vi "GetProbePlanCoordinates.vi"(8 "Use index as X coord":bool=TRUE, 9 "Probe Card Channels":i32=1) -> (0 "file path":string, 2 "OK?":bool, 3 "Array":T1(array[cluster]))   [LabVIEW 2018] (continued)
557\tX=44004.84\ty=-3214.74 \nLabel=Strip\t558\tX=44355.35\ty=-3136.62 \nLabel=Strip\t559\tX=44005.91\ty=-3067.71 \nLabel=Strip\t560\tX=44356.40\ty=-2989.46 \nLabel=Strip\t561\tX=44006.94\ty=-2920.67 \nLabel=Strip\t562\tX=44357.40\ty=-2842.30 \nLabel=Strip\t563\tX=44007.92\ty=-2773.62 \nLabel=Strip\t564\tX=44358.36\ty=-2695.14 \nLabel=Strip\t565\tX=44008.85\ty=-2626.58 \nLabel=Strip\t566\tX=44359.26\ty=-2547.98 \nLabel=Strip\t567\tX=44009.72\ty=-2479.54 \nLabel=Strip\t568\tX=44360.11\ty=-2400.81 \nLabel=Strip\t569\tX=44010.55\ty=-2332.49 \nLabel=Strip\t570\tX=44360.90\ty=-2253.65 \nLabel=Strip\t571\tX=44011.33\ty=-2185.45 \nLabel=Strip\t572\tX=44361.65\ty=-2106.48 \nLabel=Strip\t573\tX=44012.05\ty=-2038.40 \nLabel=Strip\t574\tX=44362.35\ty=-1959.31 \nLabel=Strip\t575\tX=44012.73\ty=-1891.35 \nLabel=Strip\t576\tX=44363.00\ty=-1812.14 \nLabel=Strip\t577\tX=44013.35\ty=-1744.30 \nLabel=Strip\t578\tX=44363.60\ty=-1664.97 \nLabel=Strip\t579\tX=44013.93\ty=-1597.25 \nLabel=Strip\t580\tX=44364.14\ty=-1517.80 \nLabel=Strip\t581\tX=44014.45\ty=-1450.20 \nLabel=Strip\t582\tX=44364.64\ty=-1370.62 \nLabel=Strip\t583\tX=44014.92\ty=-1303.14 \nLabel=Strip\t584\tX=44365.08\ty=-1223.45 \nLabel=Strip\t585\tX=44015.34\ty=-1156.09 \nLabel=Strip\t586\tX=44365.48\ty=-1076.27 \nLabel=Strip\t587\tX=44015.72\ty=-1009.03 \nLabel=Strip\t588\tX=44365.82\ty=-929.10 \nLabel=Strip\t589\tX=44016.04\ty=-861.97 \nLabel=Strip\t590\tX=44366.12\ty=-781.92 \nLabel=Strip\t591\tX=44016.31\ty=-714.91 \nLabel=Strip\t592\tX=44366.36\ty=-634.74 \nLabel=Strip\t593\tX=44016.53\ty=-567.86 \nLabel=Strip\t594\tX=44366.55\ty=-487.56 \nLabel=Strip\t595\tX=44016.70\ty=-420.79 \nLabel=Strip\t596\tX=44366.70\ty=-340.38 \nLabel=Strip\t597\tX=44016.82\ty=-273.73 \nLabel=Strip\t598\tX=44366.79\ty=-193.19 \nLabel=Strip\t599\tX=44016.89\ty=-126.67 \nLabel=Strip\t600\tX=44366.83\ty=-46.01 \nLabel=Strip\t601\tX=44016.90\ty=20.39 \nLabel=Strip\t602\tX=44366.82\ty=101.17 \nLabel=Strip\t603\tX=44016.87\ty=167.46 \nLabel=Strip\t604\tX=44366.76\ty=248.36 \nLabel=Strip\t605\tX=44016.79\ty=314.53 \nLabel=Strip\t606\tX=44366.65\ty=395.55 \nLabel=Strip\t607\tX=44016.66\ty=461.59 \nLabel=Strip\t608\tX=44366.49\ty=542.73 \nLabel=Strip\t609\tX=44016.47\ty=608.66 \nLabel=Strip\t610\tX=44366.28\ty=689.92 \nLabel=Strip\t611\tX=44016.24\ty=755.73 \nLabel=Strip\t612\tX=44366.01\ty=837.11 \nLabel=Strip\t613\tX=44015.95\ty=902.80 \nLabel=Strip\t614\tX=44365.70\ty=984.30 \nLabel=Strip\t615\tX=44015.62\ty=1049.87 \nLabel=Strip\t616\tX=44365.34\ty=1131.49 \nLabel=Strip\t617\tX=44015.23\ty=1196.94 \nLabel=Strip\t618\tX=44364.92\ty=1278.69 \nLabel=Strip\t619\tX=44014.80\ty=1344.01 \nLabel=Strip\t620\tX=44364.46\ty=1425.88 \nLabel=Strip\t621\tX=44014.31\ty=1491.09 \nLabel=Strip\t622\tX=44363.94\ty=1573.07 \nLabel=Strip\t623\tX=44013.77\ty=1638.16 \nLabel=Strip\t624\tX=44363.38\ty=1720.27 \nLabel=Strip\t625\tX=44013.18\ty=1785.24 \nLabel=Strip\t626\tX=44362.76\ty=1867.46 \nLabel=Strip\t627\tX=44012.55\ty=1932.31 \nLabel=Strip\t628\tX=44362.10\ty=2014.66 \nLabel=Strip\t629\tX=44011.86\ty=2079.39 \nLabel=Strip\t630\tX=44361.38\ty=2161.86 \nLabel=Strip\t631\tX=44011.12\ty=2226.47 \nLabel=Strip\t632\tX=44360.61\ty=2309.06 \nLabel=Strip\t633\tX=44010.33\ty=2373.55 \nLabel=Strip\t634\tX=44359.79\ty=2456.26 \nLabel=Strip\t635\tX=44009.49\ty=2520.63 \nLabel=Strip\t636\tX=44358.92\ty=2603.46 \nLabel=Strip\t637\tX=44008.60\ty=2667.71 \nLabel=Strip\t638\tX=44358.00\ty=2750.66 \nLabel=Strip\t639\tX=44007.65\ty=2814.79 \nLabel=Strip\t640\tX=44357.03\ty=2897.86 \nLabel=Strip\t641\tX=44006.66\ty=2961.87 \nLabel=Strip\t642\tX=44356.01\ty=3045.06 \nLabel=Strip\t643\tX=44005.62\ty=3108.95 \nLabel=Strip\t644\tX=44354.94\ty=3192.26 \nLabel=Strip\t645\tX=44004.53\ty=3256.03 \nLabel=Strip\t646\tX=44353.82\ty=3339.46 \nLabel=Strip\t647\tX=44003.38\ty=3403.12 \nLabel=Strip\t648\tX=44352.65\ty=3486.67 \nLabel=Strip\t649\tX=44002.19\ty=3550.20 \nLabel=Strip\t650\tX=44351.42\ty=3633.87 \nLabel=Strip\t651\tX=44000.94\ty=3697.28 \nLabel=Strip\t652\tX=44350.15\ty=3781.08 \nLabel=Strip\t653\tX=43999.65\ty=3844.37 \nLabel=Strip\t654\tX=44348.83\ty=3928.28 \nLabel=Strip\t655\tX=43998.30\ty=3991.46 \nLabel=Strip\t656\tX=44347.45\ty=4075.49 \nLabel=Strip\t657\tX=43996.90\ty=4138.54 \nLabel=Strip\t658\tX=44346.03\ty=4222.70 \nLabel=Strip\t659\tX=43995.46\ty=4285.63 \nLabel=Strip\t660\tX=44344.55\ty=4369.90 \nLabel=Strip\t661\tX=43993.96\ty=4432.72 \nLabel=Strip\t662\tX=44343.02\ty=4517.11 \nLabel=Strip\t663\tX=43992.41\ty=4579.80 \nLabel=Strip\t664\tX=44341.45\ty=4664.32 \nLabel=Strip\t665\tX=43990.81\ty=4726.89 \nLabel=Strip\t666\tX=44339.82\ty=4811.53 \nLabel=Strip\t667\tX=43989.16\ty=4873.98 \nLabel=Strip\t668\tX=44338.14\ty=4958.74 \nLabel=Strip\t669\tX=43987.46\ty=5021.07 \nLabel=Strip\t670\tX=44336.41\ty=5105.95 \nLabel=Strip\t671\tX=43985.71\ty=5168.16 \nLabel=Strip\t672\tX=44334.63\ty=5253.16 \nLabel=Strip\t673\tX=43983.91\ty=5315.25 \nLabel=Strip\t674\tX=44332.80\ty=5400.37 \nLabel=Strip\t675\tX=43982.06\ty=5462.34 \nLabel=Strip\t676\tX=44330.92\ty=5547.58 \nLabel=Strip\t677\tX=43980.16\ty=5609.43 \nLabel=Strip\t678\tX=44328.99\ty=5694.79 \nLabel=Strip\t679\tX=43978.21\ty=5756.52 \nLabel=Strip\t680\tX=44327.01\ty=5842.00 \nLabel=Strip\t681\tX=43976.20\ty=5903.62 \nLabel=Strip\t682\tX=44324.98\ty=5989.21 \nLabel=Strip\t683\tX=43974.15\ty=6050.71 \nLabel=Strip\t684\tX=44322.89\ty=6136.43 \nLabel=Strip\t685\tX=43972.05\ty=6197.80 \nLabel=Strip\t686\tX=44320.76\ty=6283.64 \nLabel=Strip\t687\tX=43969.89\ty=6344.89 \nLabel=Strip\t688\tX=44318.58\ty=6430.85 \nLabel=Strip\t689\tX=43967.69\ty=6491.99 \nLabel=Strip\t690\tX=44316.34\ty=6578.06 \nLabel=Strip\t691\tX=43965.43\ty=6639.08 \nLabel=Strip\t692\tX=44314.06\ty=6725.28 \nLabel=Strip\t693\tX=43963.13\ty=6786.17 \nLabel=Strip\t694\tX=44311.72\ty=6872.49 \nLabel=Strip\t695\tX=43960.77\ty=6933.27 \nLabel=Strip\t696\tX=44309.33\ty=7019.71 \nLabel=Strip\t697\tX=43958.36\ty=7080.36 \nLabel=Strip\t698\tX=44306.90\ty=7166.92 \nLabel=Strip\t699\tX=43955.90\ty=7227.45 \nLabel=Strip\t700\tX=44304.41\ty=7314.13 \nLabel=Strip\t701\tX=43953.39\ty=7374.55 \nLabel=Strip\t702\tX=44301.87\ty=7461.35 \nLabel=Strip\t703\tX=43950.84\ty=7521.64 \nLabel=Strip\t704\tX=44299.28\ty=7608.56 \nLabel=Strip\t705\tX=43948.23\ty=7668.74 \nLabel=Strip\t706\tX=44296.64\ty=7755.78 \nLabel=Strip\t707\tX=43945.57\ty=7815.83 \nLabel=Strip\t708\tX=44293.95\ty=7902.99 \nLabel=Strip\t709\tX=43942.85\ty=7962.93 \nLabel=Strip\t710\tX=44291.21\ty=8050.21 \nLabel=Strip\t711\tX=43940.09\ty=8110.02 \nLabel=Strip\t712\tX=44288.42\ty=8197.42 \nLabel=Strip\t713\tX=43937.28\ty=8257.12 \nLabel=Strip\t714\tX=44285.58\ty=8344.64 \nLabel=Strip\t715\tX=43934.42\ty=8404.21 \nLabel=Strip\t716\tX=44282.68\ty=8491.85 \nLabel=Strip\t717\tX=43931.51\ty=8551.31 \nLabel=Strip\t718\tX=44279.74\ty=8639.07 \nLabel=Strip\t719\tX=43928.54\ty=8698.40 \nLabel=Strip\t720\tX=44276.75\ty=8786.28 \nLabel=Strip\t721\tX=43925.53\ty=8845.50 \nLabel=Strip\t722\tX=44273.70\ty=8933.50 \nLabel=Strip\t723\tX=43922.46\ty=8992.59 \nLabel=Strip\t724\tX=44270.61\ty=9080.71 \nLabel=Strip\t725\tX=43919.35\ty=9139.69 \nLabel=Strip\t726\tX=44267.46\ty=9227.93 \nLabel=Strip\t727\tX=43916.18\ty=9286.78 \nLabel=Strip\t728\tX=44264.27\ty=9375.15 \nLabel=Strip\t729\tX=43912.96\ty=9433.88 \nLabel=Strip\t730\tX=44261.02\ty=9522.36 \nLabel=Strip\t731\tX=43909.70\ty=9580.97 \nLabel=Strip\t732\tX=44257.72\ty=9669.57 \nLabel=Strip\t733\tX=43906.38\ty=9728.07 \nLabel=Strip\t734\tX=44254.37\ty=9816.79 \nLabel=Strip\t735\tX=43903.01\ty=9875.16 \nLabel=Strip\t736\tX=44250.98\ty=9964.00 \nLabel=Strip\t737\tX=43899.59\ty=10022.26 \nLabel=Strip\t738\tX=44247.53\ty=10111.22 \nLabel=Strip\t739\tX=43896.12\ty=10169.35 \nLabel=Strip\t740\tX=44244.03\ty=10258.43 \nLabel=Strip\t741\tX=43892.60\ty=10316.45 \nLabel=Strip\t742\tX=44240.48\ty=10405.65 \nLabel=Strip\t743\tX=43889.03\ty=10463.54 \nLabel=Strip\t744\tX=44236.87\ty=10552.86 \nLabel=Strip\t745\tX=43885.41\ty=10610.63 \nLabel=Strip\t746\tX=44233.22\ty=10700.08 \nLabel=Strip\t747\tX=43881.74\ty=10757.73 \nLabel=Strip\t748\tX=44229.52\ty=10847.29 \nLabel=Strip\t749\tX=43878.02\ty=10904.82 \nLabel=Strip\t750\tX=44225.77\ty=10994.50 \nLabel=Strip\t751\tX=43874.25\ty=11051.91 \nLabel=Strip\t752\tX=44221.96\ty=11141.72 \nLabel=Strip\t753\tX=43870.42\ty=11199.01 \nLabel=Strip\t754\tX=44218.11\ty=11288.93 \nLabel=Strip\t755\tX=43866.55\ty=11346.10 \nLabel=Strip\t756\tX=44214.20\ty=11436.14 \nLabel=Strip\t757\tX=43862.63\ty=11493.19 \nLabel=Strip\t758\tX=44210.25\ty=11583.35 \nLabel=Strip\t759\tX=43858.65\ty=11640.28 \nLabel=Strip\t760\tX=44206.24\ty=11730.57 \nLabel=Strip\t761\tX=43854.62\ty=11787.38 \nLabel=Strip\t762\tX=44202.19\ty=11877.78 \nLabel=Strip\t763\tX=43850.55\ty=11934.47 \nLabel=Strip\t764\tX=44198.08\ty=12024.99 \nLabel=Strip\t765\tX=43846.42\ty=12081.56 \nLabel=Strip\t766\tX=44193.92\ty=12172.20 \nLabel=Strip\t767\tX=43842.24\ty=12228.65 \nLabel=Strip\t768\tX=44189.71\ty=12319.41 \nLabel=Strip\t769\tX=43838.02\ty=12375.74 \nLabel=Strip\t770\tX=44185.45\ty=12466.62 \nLabel=Strip\t771\tX=43833.74\ty=12522.83 \nLabel=Strip\t772\tX=44181.14\ty=12613.83 \nLabel=Strip\t773\tX=43829.41\ty=12669.92 \nLabel=Strip\t774\tX=44176.78\ty=12761.04 \nLabel=Strip\t775\tX=43825.03\ty=12817.01 \nLabel=Strip\t776\tX=44172.37\ty=12908.25 \nLabel=Strip\t777\tX=43820.60\ty=12964.09 \nLabel=Strip\t778\tX=44167.91\ty=13055.45 \nLabel=Strip\t779\tX=43816.12\ty=13111.18 \nLabel=Strip\t780\tX=44163.40\ty=13202.66 \nLabel=Strip\t781\tX=43811.59\ty=13258.27 \nLabel=Strip\t782\tX=44158.84\ty=13349.87 \nLabel=Strip\t783\tX=43807.00\ty=13405.36 \nLabel=Strip\t784\tX=44154.22\ty=13497.08 \nLabel=Strip\t785\tX=43802.37\ty=13552.44 \nLabel=Strip\t786\tX=44149.56\ty=13644.28 \nLabel=Strip\t787\tX=43797.69\ty=13699.53 \nLabel=Strip\t788\tX=44144.84\ty=13791.49 \nLabel=Strip\t789\tX=43792.95\ty=13846.61 \nLabel=Strip\t790\tX=44140.08\ty=13938.69 \nLabel=Strip\t791\tX=43788.17\ty=13993.70 \nLabel=Strip\t792\tX=44135.26\ty=14085.90 \nLabel=Strip\t793\tX=43783.34\ty=14140.78 \nLabel=Strip\t794\tX=44130.39\ty=14233.10 \nLabel=Strip\t795\tX=43778.45\ty=14287.87 \nLabel=Strip\t796\tX=44125.48\ty=14380.30 \nLabel=Strip\t797\tX=43773.51\ty=14434.95 \nLabel=Strip\t798\tX=44120.51\ty=14527.50 \nLabel=Strip\t799\tX=43768.53\ty=14582.03 \nLabel=Strip\t800\tX=44115.49\ty=14674.71 \nLabel=Strip\t801\tX=43763.49\ty=14729.11 \nLabel=Strip\t802\tX=44110.42\ty=14821.91 \nLabel=Strip\t803\tX=43758.40\ty=14876.19 \nLabel=Strip\t804\tX=44105.30\ty=14969.11 \nLabel=Strip\t805\tX=43753.26\ty=15023.27 \nLabel=Strip\t806\tX=44100.13\ty=15116.31 \nLabel=Strip\t807\tX=43748.07\ty=15170.35 \nLabel=Strip\t808\tX=44094.91\ty=15263.50 \nLabel=Strip\t809\tX=43742.83\ty=15317.43 \nLabel=Strip\t810\tX=44089.64\ty=15410.70 \nLabel=Strip\t811\tX=43737.54\ty=15464.51 \nLabel=Strip\t812\tX=44084.32\ty=15557.90 \nLabel=Strip\t813\tX=43732.20\ty=15611.58 \nLabel=Strip\t814\tX=44078.94\ty=15705.10 \nLabel=Strip\t815\tX=43726.81\ty=15758.66 \nLabel=Strip\t816\tX=44073.52\ty=15852.29 \nLabel=Strip\t817\tX=43721.37\ty=15905.73 \nLabel=Strip\t818\tX=44068.05\ty=15999.49 \nLabel=Strip\t819\tX=43715.88\ty=16052.81 \nLabel=Strip\t820\tX=44062.52\ty=16146.68 \nLabel=Strip\t821\tX=43710.33\ty=16199.88 \nLabel=Strip\t822\tX=44056.95\ty=16293.87 \nLabel=Strip\t823\tX=43704.74\ty=16346.95 \nLabel=Strip\t824\tX=44051.32\ty=16441.06 \nLabel=Strip\t825\tX=43699.10\ty=16494.02 \nLabel=Strip\t826\tX=44045.64\ty=16588.26 \nLabel=Strip\t827\tX=43693.40\ty=16641.10 \nLabel=Strip\t828\tX=44039.92\ty=16735.44 \nLabel=Strip\t829\tX=43687.66\ty=16788.17 \nLabel=Strip\t830\tX=44034.14\ty=16882.63 \nLabel=Strip\t831\tX=43681.86\ty=16935.23 \nLabel=Strip\t832\tX=44028.31\ty=17029.82 \nLabel=Strip\t833\tX=43676.01\ty=17082.30 \nLabel=Strip\t834\tX=44022.43\ty=17177.01 \nLabel=Strip\t835\tX=43670.12\ty=17229.37 \nLabel=Strip\t836\tX=44016.50\ty=17324.20 \nLabel=Strip\t837\tX=43664.17\ty=17376.43 \nLabel=Strip\t838\tX=44010.52\ty=17471.38 \nLabel=Strip\t839\tX=43658.17\ty=17523.50 \nLabel=Strip\t840\tX=44004.49\ty=17618.57 \nLabel=Strip\t841\tX=43652.12\ty=17670.56 \nLabel=Strip\t842\tX=43998.41\ty=17765.75 \nLabel=Strip\t843\tX=43646.02\ty=17817.62 \nLabel=Strip\t844\tX=43992.27\ty=17912.93 \nLabel=Strip\t845\tX=43639.87\ty=17964.69 \nLabel=Strip\t846\tX=43986.09\ty=18060.11 \nLabel=Strip\t847\tX=43633.67\ty=18111.75 \nLabel=Strip\t848\tX=43979.86\ty=18207.29 \nLabel=Strip\t849\tX=43627.42\ty=18258.81 \nLabel=Strip\t850\tX=43973.57\ty=18354.47 \nLabel=Strip\t851\tX=43621.11\ty=18405.86 \nLabel=Strip\t852\tX=43967.24\ty=18501.65 \nLabel=Strip\t853\tX=43614.76\ty=18552.92 \nLabel=Strip\t854\tX=43960.85\ty=18648.82 \nLabel=Strip\t855\tX=43608.36\ty=18699.98 \nLabel=Strip\t856\tX=43954.41\ty=18796.00 \nLabel=Strip\t857\tX=43601.90\ty=18847.03 \nLabel=Strip\t858\tX=43947.93\ty=18943.17 \nLabel=Strip\t859\tX=43595.40\ty=18994.09 \nLabel=Strip\t860\tX=43941.39\ty=19090.35 \nLabel=Strip\t861\tX=43588.84\ty=19141.14 \nLabel=Strip\t862\tX=43934.80\ty=19237.52 \nLabel=Strip\t863\tX=43582.24\ty=19288.19 \nLabel=Strip\t864\tX=43928.16\ty=19384.69 \nLabel=Strip\t865\tX=43575.58\ty=19435.24 \nLabel=Strip\t866\tX=43921.47\ty=19531.86 \nLabel=Strip\t867\tX=43568.88\ty=19582.29 \nLabel=Strip\t868\tX=43914.73\ty=19679.03 \nLabel=Strip\t869\tX=43562.12\ty=19729.34 \nLabel=Strip\t870\tX=43907.94\ty=19826.19 \nLabel=Strip\t871\tX=43555.31\ty=19876.38 \nLabel=Strip\t872\tX=43901.10\ty=19973.36 \nLabel=Strip\t873\tX=43548.45\ty=20023.43 \nLabel=Strip\t874\tX=43894.21\ty=20120.52 \nLabel=Strip\t875\tX=43541.54\ty=20170.47 \nLabel=Strip\t876\tX=43887.26\ty=20267.68 \nLabel=Strip\t877\tX=43534.58\ty=20317.51 \nLabel=Strip\t878\tX=43880.27\ty=20414.85 \nLabel=Strip\t879\tX=43527.57\ty=20464.55 \nLabel=Strip\t880\tX=43873.23\ty=20562.01 \nLabel=Strip\t881\tX=43520.51\ty=20611.59 \nLabel=Strip\t882\tX=43866.13\ty=20709.16 \nLabel=Strip\t883\tX=43513.40\ty=20758.63 \nLabel=Strip\t884\tX=43858.99\ty=20856.32 \nLabel=Strip\t885\tX=43506.24\ty=20905.67 \nLabel=Strip\t886\tX=43851.79\ty=21003.48 \nLabel=Strip\t887\tX=43499.02\ty=21052.70 \nLabel=Strip\t888\tX=43844.55\ty=21150.63 \nLabel=Strip\t889\tX=43491.76\ty=21199.73 \nLabel=Strip\t890\tX=43837.25\ty=21297.78 \nLabel=Strip\t891\tX=43484.45\ty=21346.77 \nLabel=Strip\t892\tX=43829.90\ty=21444.93 \nLabel=Strip\t893\tX=43477.08\ty=21493.80 \nLabel=Strip\t894\tX=43822.50\ty=21592.08 \nLabel=Strip\t895\tX=43469.66\ty=21640.83 \nLabel=Strip\t896\tX=43815.05\ty=21739.23 \nLabel=Strip\t897\tX=43462.20\ty=21787.85 \nLabel=Strip\t898\tX=43807.55\ty=21886.38 \nLabel=Strip\t899\tX=43454.68\ty=21934.88 \nLabel=Strip\t900\tX=43800.00\ty=22033.52 \nLabel=Strip\t901\tX=43447.12\ty=22081.90 \nLabel=Strip\t902\tX=43792.40\ty=22180.67 \nLabel=Strip\t903\tX=43439.50\ty=22228.93 \nLabel=Strip\t904\tX=43784.75\ty=22327.81 \nLabel=Strip\t905\tX=43431.83\ty=22375.95 \nLabel=Strip\t906\tX=43777.05\ty=22474.95 \nLabel=Strip\t907\tX=43424.11\ty=22522.97 \nLabel=Strip\t908\tX=43769.29\ty=22622.09 \nLabel=Strip\t909\tX=43416.34\ty=22669.99 \nLabel=Strip\t910\tX=43761.49\ty=22769.23 \nLabel=Strip\t911\tX=43408.52\ty=22817.00 \nLabel=Strip\t912\tX=43753.63\ty=22916.36 \nLabel=Strip\t913\tX=43400.65\ty=22964.02 \nLabel=Strip\t914\tX=43745.73\ty=23063.49 \nLabel=Strip\t915\tX=43392.73\ty=23111.03 \nLabel=Strip\t916\tX=43737.77\ty=23210.63 \nLabel=Strip\t917\tX=43384.76\ty=23258.04 \nLabel=Strip\t918\tX=43729.77\ty=23357.76 \nLabel=Strip\t919\tX=43376.73\ty=23405.05 \nLabel=Strip\t920\tX=43721.71\ty=23504.89 \nLabel=Strip\t921\tX=43368.66\ty=23552.06 \nLabel=Strip\t922\tX=43713.60\ty=23652.01 \nLabel=Strip\t923\tX=43360.54\ty=23699.06 \nLabel=Strip\t924\tX=43705.44\ty=23799.14 \nLabel=Strip\t925\tX=43352.36\ty=23846.07 \nLabel=Strip\t926\tX=43697.24\ty=23946.26 \nLabel=Strip\t927\tX=43344.14\ty=23993.07 \nLabel=Strip\t928\tX=43688.98\ty=24093.38 \nLabel=Strip\t929\tX=43335.86\ty=24140.07 \nLabel=Strip\t930\tX=43680.67\ty=24240.50 \nLabel=Strip\t931\tX=43327.53\ty=24287.07 \nLabel=Strip\t932\tX=43672.30\ty=24387.62 \nLabel=Strip\t933\tX=43319.16\ty=24434.07 \nLabel=Strip\t934\tX=43663.89\ty=24534.74 \nLabel=Strip\t935\tX=43310.73\ty=24581.06 \nLabel=Strip\t936\tX=43655.43\ty=24681.85 \nLabel=Strip\t937\tX=43302.25\ty=24728.06 \nLabel=Strip\t938\tX=43646.92\ty=24828.96 \nLabel=Strip\t939\tX=43293.72\ty=24875.05 \nLabel=Strip\t940\tX=43638.35\ty=24976.07 \nLabel=Strip\t941\tX=43285.14\ty=25022.04 \nLabel=Strip\t942\tX=43629.74\ty=25123.18 \nLabel=Strip\t943\tX=43276.51\ty=25169.02 \nLabel=Strip\t944\tX=43621.08\ty=25270.29 \nLabel=Strip\t945\tX=43267.83\ty=25316.01 \nLabel=Strip\t946\tX=43612.36\ty=25417.39 \nLabel=Strip\t947\tX=43259.10\ty=25462.99 \nLabel=Strip\t948\tX=43603.59\ty=25564.49 \nLabel=Strip\t949\tX=43250.32\ty=25609.98 \nLabel=Strip\t950\tX=43594.78\ty=25711.59 \nLabel=Strip\t951\tX=43241.49\ty=25756.96 \nLabel=Strip\t952\tX=43585.91\ty=25858.69 \nLabel=Strip\t953\tX=43232.60\ty=25903.93 \nLabel=Strip\t954\tX=43576.99\ty=26005.79 \nLabel=Strip\t955\tX=43223.67\ty=26050.91 \nLabel=Strip\t956\tX=43568.02\ty=26152.88 \nLabel=Strip\t957\tX=43214.69\ty=26197.88 \nLabel=Strip\t958\tX=43559.00\ty=26299.98 \nLabel=Strip\t959\tX=43205.65\ty=26344.85 \nLabel=Strip\t960\tX=43549.93\ty=26447.07 \nLabel=Strip\t961\tX=43196.57\ty=26491.82 \nLabel=Strip\t962\tX=43540.81\ty=26594.15 \nLabel=Strip\t963\tX=43187.43\ty=26638.79 \nLabel=Strip\t964\tX=43531.64\ty=26741.24 \nLabel=Strip\t965\tX=43178.24\ty=26785.76 \nLabel=Strip\t966\tX=43522.42\ty=26888.32 \nLabel=Strip\t967\tX=43169.01\ty=26932.72 \nLabel=Strip\t968\tX=43513.15\ty=27035.41 \nLabel=Strip\t969\tX=43159.72\ty=27079.68 \nLabel=Strip\t970\tX=43503.82\ty=27182.49 \nLabel=Strip\t971\tX=43150.38\ty=27226.64 \nLabel=Strip\t972\tX=43494.45\ty=27329.56 \nLabel=Strip\t973\tX=43140.99\ty=27373.59 \nLabel=Strip\t974\tX=43485.03\ty=27476.64 \nLabel=Strip\t975\tX=43131.55\ty=27520.55 \nLabel=Strip\t976\tX=43475.55\ty=27623.71 \nLabel=Strip\t977\tX=43122.06\ty=27667.50 \nLabel=Strip\t978\tX=43466.03\ty=27770.78 \nLabel=Strip\t979\tX=43112.52\ty=27814.45 \nLabel=Strip\t980\tX=43456.45\ty=27917.85 \nLabel=Strip\t981\tX=43102.93\ty=27961.40 \nLabel=Strip\t982\tX=43446.82\ty=28064.92 \nLabel=Strip\t983\tX=43093.29\ty=28108.34 \nLabel=Strip\t984\tX=43437.14\ty=28211.98 \nLabel=Strip\t985\tX=43083.59\ty=28255.29 \nLabel=Strip\t986\tX=43427.41\ty=28359.04 \nLabel=Strip\t987\tX=43073.85\ty=28402.23 \nLabel=Strip\t988\tX=43417.64\ty=28506.10 \nLabel=Strip\t989\tX=43064.06\ty=28549.17 \nLabel=Strip\t990\tX=43407.81\ty=28653.16 \nLabel=Strip\t991\tX=43054.21\ty=28696.10 \nLabel=Strip\t992\tX=43397.93\ty=28800.21 \nLabel=Strip\t993\tX=43044.32\ty=28843.04 \nLabel=Strip\t994\tX=43388.00\ty=28947.26 \nLabel=Strip\t995\tX=43034.37\ty=28989.97 \nLabel=Strip\t996\tX=43378.01\ty=29094.31 \nLabel=Strip\t997\tX=43024.37\ty=29136.90 \nLabel=Strip\t998\tX=43367.98\ty=29241.36 \nLabel=Strip\t999\tX=43014.33\ty=29283.82 \nLabel=Strip\t1000\tX=43357.90\ty=29388.41 \nLabel=Strip\t1001\tX=43004.23\ty=29430.75 \nLabel=Strip\t1002\tX=43347.76\ty=29535.45 \nLabel=Strip\t1003\tX=42994.08\ty=29577.67 \nLabel=Strip\t1004\tX=43337.58\ty=29682.49 \nLabel=Strip\t1005\tX=42983.88\ty=29724.59 \nLabel=Strip\t1006\tX=43327.35\ty=29829.53 \nLabel=Strip\t1007\tX=42973.63\ty=29871.50 \nLabel=Strip\t1008\tX=43317.06\ty=29976.56 \nLabel=Strip\t1009\tX=42963.33\ty=30018.42 \nLabel=Strip\t1010\tX=43306.72\ty=30123.60 \nLabel=Strip\t1011\tX=42952.98\ty=30165.33 \nLabel=Strip\t1012\tX=43296.34\ty=30270.63 \nLabel=Strip\t1013\tX=42942.58\ty=30312.24 \nLabel=Strip\t1014\tX=43285.90\ty=30417.65 \nLabel=Strip\t1015\tX=42932.13\ty=30459.15 \nLabel=Strip\t1016\tX=43275.41\ty=30564.68 \nLabel=Strip\t1017\tX=42921.63\ty=30606.05 \nLabel=Strip\t1018\tX=43264.87\ty=30711.70 \nLabel=Strip\t1019\tX=42911.07\ty=30752.95 \nLabel=Strip\t1020\tX=43254.28\ty=30858.72 \nLabel=Strip\t1021\tX=42900.47\ty=30899.85 \nLabel=Strip\t1022\tX=43243.64\ty=31005.74 \nLabel=Strip\t1023\tX=42889.82\ty=31046.75 \nLabel=Strip\t1024\tX=43232.95\ty=31152.75 \nLabel=Strip\t1025\tX=42879.11\ty=31193.64 \nLabel=Strip\t1026\tX=43222.21\ty=31299.76 \nLabel=Strip\t1027\tX=42868.36\ty=31340.53 \nLabel=Strip\t1028\tX=43211.42\ty=31446.77 \nLabel=Strip\t1029\tX=42857.55\ty=31487.42 \nLabel=Strip\t1030\tX=43200.58\ty=31593.78 \nLabel=Strip\t1031\tX=42846.69\ty=31634.30 \nLabel=Strip\t1032\tX=43189.68\ty=31740.78 \nLabel=Strip\t1033\tX=42835.79\ty=31781.19 \nLabel=Strip\t1034\tX=43178.74\ty=31887.78 \nLabel=Strip\t1035\tX=42824.83\ty=31928.07 \nLabel=Strip\t1036\tX=43167.74\ty=32034.78 \nLabel=Strip\t1037\tX=42813.82\ty=32074.94 \nLabel=Strip\t1038\tX=43156.70\ty=32181.78 \nLabel=Strip\t1039\tX=42802.76\ty=32221.82 \nLabel=Strip\t1040\tX=43145.60\ty=32328.77 \nLabel=Strip\t1041\tX=42791.65\ty=32368.69 \nLabel=Strip\t1042\tX=43134.46\ty=32475.76 \nLabel=Strip\t1043\tX=42780.49\ty=32515.56 \nLabel=Strip\t1044\tX=43123.26\ty=32622.75 \nLabel=Strip\t1045\tX=42769.28\ty=32662.42 \nLabel=Strip\t1046\tX=43112.01\ty=32769.73 \nLabel=Strip\t1047\tX=42758.02\ty=32809.29 \nLabel=Strip\t1048\tX=43100.71\ty=32916.71 \nLabel=Strip\t1049\tX=42746.71\ty=32956.15 \nLabel=Strip\t1050\tX=43089.36\ty=33063.69 \nLabel=Strip\t1051\tX=42735.34\ty=33103.01 \nLabel=Strip\t1052\tX=43077.97\ty=33210.67 \nLabel=Strip\t1053\tX=42723.93\ty=33249.86 \nLabel=Strip\t1054\tX=43066.51\ty=33357.64 \nLabel=Strip\t1055\tX=42712.47\ty=33396.71 \nLabel=Strip\t1056\tX=43055.01\ty=33504.61 \nLabel=Strip\t1057\tX=42700.95\ty=33543.56 \nLabel=Strip\t1058\tX=43043.46\ty=33651.58 \nLabel=Strip\t1059\tX=42689.39\ty=33690.41 \nLabel=Strip\t1060\tX=43031.86\ty=33798.54 \nLabel=Strip\t1061\tX=42677.77\ty=33837.25 \nLabel=Strip\t1062\tX=43020.21\ty=33945.50 \nLabel=Strip\t1063\tX=42666.11\ty=33984.09 \nLabel=Strip\t1064\tX=43008.50\ty=34092.46 \nLabel=Strip\t1065\tX=42654.39\ty=34130.93 \nLabel=Strip\t1066\tX=42996.75\ty=34239.41 \nLabel=Strip\t1067\tX=42642.62\ty=34277.76 \nLabel=Strip\t1068\tX=42984.94\ty=34386.37 \nLabel=Strip\t1069\tX=42630.80\ty=34424.59 \nLabel=Strip\t1070\tX=42973.09\ty=34533.31 \nLabel=Strip\t1071\tX=42618.93\ty=34571.42 \nLabel=Strip\t1072\tX=42961.18\ty=34680.26 \nLabel=Strip\t1073\tX=42607.01\ty=34718.24 \nLabel=Strip\t1074\tX=42949.23\ty=34827.20 \nLabel=Strip\t1075\tX=42595.05\ty=34865.06 \nLabel=Strip\t1076\tX=42937.22\ty=34974.14 \nLabel=Strip\t1077\tX=42583.02\ty=35011.88 \nLabel=Strip\t1078\tX=42925.16\ty=35121.08 \nLabel=Strip\t1079\tX=42570.95\ty=35158.70 \nLabel=Strip\t1080\tX=42913.05\ty=35268.01 \nLabel=Strip\t1081\tX=42558.83\ty=35305.51 \nLabel=Strip\t1082\tX=42900.89\ty=35414.94 \nLabel=Strip\t1083\tX=42546.66\ty=35452.32 \nLabel=Strip\t1084\tX=42888.68\ty=35561.87 \nLabel=Strip\t1085\tX=42534.44\ty=35599.13 \nLabel=Strip\t1086\tX=42876.42\ty=35708.79 \nLabel=Strip\t1087\tX=42522.16\ty=35745.93 \nLabel=Strip\t1088\tX=42864.11\ty=35855.71 \nLabel=Strip\t1089\tX=42509.84\ty=35892.73 \nLabel=Strip\t1090\tX=42851.75\ty=36002.63 \nLabel=Strip\t1091\tX=42497.46\ty=36039.52 \nLabel=Strip\t1092\tX=42839.34\ty=36149.55 \nLabel=Strip\t1093\tX=42485.04\ty=36186.32 \nLabel=Strip\t1094\tX=42826.87\ty=36296.46 \nLabel=Strip\t1095\tX=42472.56\ty=36333.11 \nLabel=Strip\t1096\tX=42814.36\ty=36443.36 \nLabel=Strip\t1097\tX=42460.04\ty=36479.89 \nLabel=Strip\t1098\tX=42801.80\ty=36590.27 \nLabel=Strip\t1099\tX=42447.46\ty=36626.68 \nLabel=Strip\t1100\tX=42789.18\ty=36737.17 \nLabel=Strip\t1101\tX=42434.83\ty=36773.46 \nLabel=Strip\t1102\tX=42776.52\ty=36884.07 \nLabel=Strip\t1103\tX=42422.15\ty=36920.23 \nLabel=Strip\t1104\tX=42763.80\ty=37030.96 \nLabel=Strip\t1105\tX=42409.43\ty=37067.01 \nLabel=Strip\t1106\tX=42751.03\ty=37177.85 \nLabel=Strip\t1107\tX=42396.65\ty=37213.78 \nLabel=Strip\t1108\tX=42738.21\ty=37324.74 \nLabel=Strip\t1109\tX=42383.82\ty=37360.54 \nLabel=Strip\t1110\tX=42725.35\ty=37471.63 \nLabel=Strip\t1111\tX=42370.94\ty=37507.31 \nLabel=Strip\t1112\tX=42712.43\ty=37618.51 \nLabel=Strip\t1113\tX=42358.00\ty=37654.07 \nLabel=Strip\t1114\tX=42699.46\ty=37765.38 \nLabel=Strip\t1115\tX=42345.02\ty=37800.82 \nLabel=Strip\t1116\tX=42686.44\ty=37912.26 \nLabel=Strip\t1117\tX=42331.99\ty=37947.58 \nLabel=Strip\t1118\tX=42673.37\ty=38059.13 \nLabel=Strip\t1119\tX=42318.91\ty=38094.32 \nLabel=Strip\t1120\tX=42660.25\ty=38206.00 \nLabel=Strip\t1121\tX=42305.77\ty=38241.07 \nLabel=Strip\t1122\tX=42647.07\ty=38352.86 \nLabel=Strip\t1123\tX=42292.59\ty=38387.81 \nLabel=Strip\t1124\tX=42633.85\ty=38499.72 \nLabel=Strip\t1125\tX=42279.36\ty=38534.55 \nLabel=Strip\t1126\tX=42620.58\ty=38646.58 \nLabel=Strip\t1127\tX=42266.07\ty=38681.29 \nLabel=Strip\t1128\tX=42607.25\ty=38793.43 \nLabel=Strip\t1129\tX=42252.73\ty=38828.02 \nLabel=Strip\t1130\tX=42593.88\ty=38940.28 \nLabel=Strip\t1131\tX=42239.35\ty=38974.75 \nLabel=Strip\t1132\tX=42580.45\ty=39087.12 \nLabel=Strip\t1133\tX=42225.91\ty=39121.47 \nLabel=Strip\t1134\tX=42566.98\ty=39233.97 \nLabel=Strip\t1135\tX=42212.42\ty=39268.19 \nLabel=Strip\t1136\tX=42553.45\ty=39380.80 \nLabel=Strip\t1137\tX=42198.89\ty=39414.91 \nLabel=Strip\t1138\tX=42539.88\ty=39527.64 \nLabel=Strip\t1139\tX=42185.30\ty=39561.62 \nLabel=Strip\t1140\tX=42526.25\ty=39674.47 \nLabel=Strip\t1141\tX=42171.66\ty=39708.33 \nLabel=Strip\t1142\tX=42512.57\ty=39821.30 \nLabel=Strip\t1143\tX=42157.97\ty=39855.04 \nLabel=Strip\t1144\tX=42498.84\ty=39968.12 \nLabel=Strip\t1145\tX=42144.23\ty=40001.74 \nLabel=Strip\t1146\tX=42485.06\ty=40114.94 \nLabel=Strip\t1147\tX=42130.44\ty=40148.44 \nLabel=Strip\t1148\tX=42471.23\ty=40261.76 \nLabel=Strip\t1149\tX=42116.59\ty=40295.14 \nLabel=Strip\t1150\tX=42457.35\ty=40408.57 \nLabel=Strip\t1151\tX=42102.70\ty=40441.83 \nLabel=Strip\t1152\tX=42443.42\ty=40555.38 \nLabel=Strip\t1153\tX=42088.76\ty=40588.52 \nLabel=Strip\t1154\tX=42429.44\ty=40702.19 \nRegion=Segment\t1B\nLabel=Strip\t1\tX=69143.27\ty=-46239.02 \nLabel=Strip\t2\tX=69500.01\ty=-46190.10 \nLabel=Strip\t3\tX=69159.10\ty=-46083.63 \nLabel=Strip\t4\tX=69515.81\ty=-46034.59 \nLabel=Strip\t5\tX=69174.87\ty=-45928.24 \nLabel=Strip\t6\tX=69531.57\ty=-45879.07 \nLabel=Strip\t7\tX=69190.58\ty=-45772.84 \nLabel=Strip\t8\tX=69547.27\ty=-45723.55 \nLabel=Strip\t9\tX=69206.25\ty=-45617.43 \nLabel=Strip\t10\tX=69562.91\ty=-45568.02 \nLabel=Strip\t11\tX=69221.86\ty=-45462.02 \nLabel=Strip\t12\tX=69578.51\ty=-45412.49 \nLabel=Strip\t13\tX=69237.42\ty=-45306.60 \nLabel=Strip\t14\tX=69594.05\ty=-45256.94 \nLabel=Strip\t15\tX=69252.92\ty=-45151.17 \nLabel=Strip\t16\tX=69609.54\ty=-45101.39 \nLabel=Strip\t17\tX=69268.37\ty=-44995.74 \nLabel=Strip\t18\tX=69624.97\ty=-44945.84 \nLabel=Strip\t19\tX=69283.77\ty=-44840.30 \nLabel=Strip\t20\tX=69640.35\ty=-44790.28 \nLabel=Strip\t21\tX=69299.11\ty=-44684.86 \nLabel=Strip\t22\tX=69655.68\ty=-44634.71 \nLabel=Strip\t23\tX=69314.41\ty=-44529.41 \nLabel=Strip\t24\tX=69670.95\ty=-44479.14 \nLabel=Strip\t25\tX=69329.64\ty=-44373.95 \nLabel=Strip\t26\tX=69686.17\ty=-44323.56 \nLabel=Strip\t27\tX=69344.83\ty=-44218.49 \nLabel=Strip\t28\tX=69701.34\ty=-44167.97 \nLabel=Strip\t29\tX=69359.96\ty=-44063.02 \nLabel=Strip\t30\tX=69716.46\ty=-44012.38 \nLabel=Strip\t31\tX=69375.04\ty=-43907.54 \nLabel=Strip\t32\tX=69731.52\ty=-43856.78 \nLabel=Strip\t33\tX=69390.07\ty=-43752.06 \nLabel=Strip\t34\tX=69746.53\ty=-43701.18 \nLabel=Strip\t35\tX=69405.04\ty=-43596.58 \nLabel=Strip\t36\tX=69761.48\ty=-43545.57 \nLabel=Strip\t37\tX=69419.96\ty=-43441.08 \nLabel=Strip\t38\tX=69776.38\ty=-43389.96 \nLabel=Strip\t39\tX=69434.82\ty=-43285.58 \nLabel=Strip\t40\tX=69791.23\ty=-43234.33 \nLabel=Strip\t41\tX=69449.64\ty=-43130.08 \nLabel=Strip\t42\tX=69806.03\ty=-43078.70 \nLabel=Strip\t43\tX=69464.40\ty=-42974.56 \nLabel=Strip\t44\tX=69820.77\ty=-42923.06 \nLabel=Strip\t45\tX=69479.10\ty=-42819.04 \nLabel=Strip\t46\tX=69835.46\ty=-42767.42 \nLabel=Strip\t47\tX=69493.75\ty=-42663.52 \nLabel=Strip\t48\tX=69850.09\ty=-42611.77 \nLabel=Strip\t49\tX=69508.35\ty=-42507.99 \nLabel=Strip\t50\tX=69864.68\ty=-42456.12 \nLabel=Strip\t51\tX=69522.90\ty=-42352.45 \nLabel=Strip\t52\tX=69879.20\ty=-42300.46 \nLabel=Strip\t53\tX=69537.39\ty=-42196.91 \nLabel=Strip\t54\tX=69893.68\ty=-42144.80 \nLabel=Strip\t55\tX=69551.84\ty=-42041.36 \nLabel=Strip\t56\tX=69908.10\ty=-41989.13 \nLabel=Strip\t57\tX=69566.22\ty=-41885.81 \nLabel=Strip\t58\tX=69922.47\ty=-41833.45 \nLabel=Strip\t59\tX=69580.56\ty=-41730.25 \nLabel=Strip\t60\tX=69936.79\ty=-41677.76 \nLabel=Strip\t61\tX=69594.84\ty=-41574.68 \nLabel=Strip\t62\tX=69951.05\ty=-41522.08 \nLabel=Strip\t63\tX=69609.06\ty=-41419.11 \nLabel=Strip\t64\tX=69965.26\ty=-41366.38 \nLabel=Strip\t65\tX=69623.24\ty=-41263.53 \nLabel=Strip\t66\tX=69979.41\ty=-41210.68 \nLabel=Strip\t67\tX=69637.36\ty=-41107.95 \nLabel=Strip\t68\tX=69993.52\ty=-41054.97 \nLabel=Strip\t69\tX=69651.43\ty=-40952.36 \nLabel=Strip\t70\tX=70007.57\ty=-40899.26 \nLabel=Strip\t71\tX=69665.44\ty=-40796.76 \nLabel=Strip\t72\tX=70021.56\ty=-40743.54 \nLabel=Strip\t73\tX=69679.40\ty=-40641.16 \nLabel=Strip\t74\tX=70035.51\ty=-40587.82 \nLabel=Strip\t75\tX=69693.31\ty=-40485.55 \nLabel=Strip\t76\tX=70049.39\ty=-40432.09 \nLabel=Strip\t77\tX=69707.16\ty=-40329.94 \nLabel=Strip\t78\tX=70063.23\ty=-40276.35 \nLabel=Strip\t79\tX=69720.96\ty=-40174.32 \nLabel=Strip\t80\tX=70077.01\ty=-40120.61 \nLabel=Strip\t81\tX=69734.71\ty=-40018.70 \nLabel=Strip\t82\tX=70090.74\ty=-39964.86 \nLabel=Strip\t83\tX=69748.41\ty=-39863.06 \nLabel=Strip\t84\tX=70104.42\ty=-39809.11 \nLabel=Strip\t85\tX=69762.05\ty=-39707.43 \nLabel=Strip\t86\tX=70118.04\ty=-39653.35 \nLabel=Strip\t87\tX=69775.64\ty=-39551.79 \nLabel=Strip\t88\tX=70131.61\ty=-39497.58 \nLabel=Strip\t89\tX=69789.17\ty=-39396.14 \nLabel=Strip\t90\tX=70145.13\ty=-39341.82 \nLabel=Strip\t91\tX=69802.65\ty=-39240.49 \nLabel=Strip\t92\tX=70158.59\ty=-39186.04 \nLabel=Strip\t93\tX=69816.08\ty=-39084.83 \nLabel=Strip\t94\tX=70172.00\ty=-39030.26 \nLabel=Strip\t95\tX=69829.46\ty=-38929.16 \nLabel=Strip\t96\tX=70185.36\ty=-38874.47 \nLabel=Strip\t97\tX=69842.78\ty=-38773.49 \nLabel=Strip\t98\tX=70198.66\ty=-38718.68 \nLabel=Strip\t99\tX=69856.05\ty=-38617.82 \nLabel=Strip\t100\tX=70211.91\ty=-38562.88 \nLabel=Strip\t101\tX=69869.26\ty=-38462.14 \nLabel=Strip\t102\tX=70225.11\ty=-38407.08 \nLabel=Strip\t103\tX=69882.42\ty=-38306.45 \nLabel=Strip\t104\tX=70238.25\ty=-38251.27 \nLabel=Strip\t105\tX=69895.53\ty=-38150.76 \nLabel=Strip\t106\tX=70251.34\ty=-38095.45 \nLabel=Strip\t107\tX=69908.59\ty=-37995.06 \nLabel=Strip\t108\tX=70264.38\ty=-37939.63 \nLabel=Strip\t109\tX=69921.59\ty=-37839.36 \nLabel=Strip\t110\tX=70277.36\ty=-37783.80 \nLabel=Strip\t111\tX=69934.54\ty=-37683.65 \nLabel=Strip\t112\tX=70290.29\ty=-37627.97 \nLabel=Strip\t113\tX=69947.43\ty=-37527.93 \nLabel=Strip\t114\tX=70303.16\ty=-37472.14 \nLabel=Strip\t115\tX=69960.27\ty=-37372.21 \nLabel=Strip\t116\tX=70315.99\ty=-37316.29 \nLabel=Strip\t117\tX=69973.06\ty=-37216.49 \nLabel=Strip\t118\tX=70328.76\ty=-37160.45 \nLabel=Strip\t119\tX=69985.80\ty=-37060.76 \nLabel=Strip\t120\tX=70341.47\ty=-37004.59 \nLabel=Strip\t121\tX=69998.48\ty=-36905.02 \nLabel=Strip\t122\tX=70354.14\ty=-36848.73 \nLabel=Strip\t123\tX=70011.11\ty=-36749.28 \nLabel=Strip\t124\tX=70366.75\ty=-36692.87 \nLabel=Strip\t125\tX=70023.68\ty=-36593.53 \nLabel=Strip\t126\tX=70379.30\ty=-36537.00 \nLabel=Strip\t127\tX=70036.21\ty=-36437.78 \nLabel=Strip\t128\tX=70391.80\ty=-36381.13 \nLabel=Strip\t129\tX=70048.68\ty=-36282.02 \nLabel=Strip\t130\tX=70404.25\ty=-36225.25 \nLabel=Strip\t131\tX=70061.09\ty=-36126.26 \nLabel=Strip\t132\tX=70416.65\ty=-36069.36 \nLabel=Strip\t133\tX=70073.45\ty=-35970.50 \nLabel=Strip\t134\tX=70428.99\ty=-35913.47 \nLabel=Strip\t135\tX=70085.76\ty=-35814.72 \nLabel=Strip\t136\tX=70441.28\ty=-35757.58 \nLabel=Strip\t137\tX=70098.02\ty=-35658.94 \nLabel=Strip\t138\tX=70453.52\ty=-35601.68 \nLabel=Strip\t139\tX=70110.22\ty=-35503.16 \nLabel=Strip\t140\tX=70465.70\ty=-35445.77 \nLabel=Strip\t141\tX=70122.37\ty=-35347.37 \nLabel=Strip\t142\tX=70477.83\ty=-35289.86 \nLabel=Strip\t143\tX=70134.46\ty=-35191.58 \nLabel=Strip\t144\tX=70489.90\ty=-35133.94 \nLabel=Strip\t145\tX=70146.51\ty=-35035.78 \nLabel=Strip\t146\tX=70501.93\ty=-34978.02 \nLabel=Strip\t147\tX=70158.49\ty=-34879.97 \nLabel=Strip\t148\tX=70513.90\ty=-34822.09 \nLabel=Strip\t149\tX=70170.43\ty=-34724.16 \nLabel=Strip\t150\tX=70525.81\ty=-34666.16 \nLabel=Strip\t151\tX=70182.31\ty=-34568.35 \nLabel=Strip\t152\tX=70537.67\ty=-34510.22 \nLabel=Strip\t153\tX=70194.14\ty=-34412.53 \nLabel=Strip\t154\tX=70549.48\ty=-34354.28 \nLabel=Strip\t155\tX=70205.92\ty=-34256.71 \nLabel=Strip\t156\tX=70561.24\ty=-34198.33 \nLabel=Strip\t157\tX=70217.64\ty=-34100.88 \nLabel=Strip\t158\tX=70572.94\ty=-34042.38 \nLabel=Strip\t159\tX=70229.31\ty=-33945.04 \nLabel=Strip\t160\tX=70584.59\ty=-33886.43 \nLabel=Strip\t161\tX=70240.92\ty=-33789.20 \nLabel=Strip\t162\tX=70596.18\ty=-33730.46 \nLabel=Strip\t163\tX=70252.48\ty=-33633.36 \nLabel=Strip\t164\tX=70607.72\ty=-33574.50 \nLabel=Strip\t165\tX=70263.99\ty=-33477.51 \nLabel=Strip\t166\tX=70619.21\ty=-33418.52 \nLabel=Strip\t167\tX=70275.45\ty=-33321.65 \nLabel=Strip\t168\tX=70630.65\ty=-33262.55 \nLabel=Strip\t169\tX=70286.85\ty=-33165.79 \nLabel=Strip\t170\tX=70642.03\ty=-33106.56 \nLabel=Strip\t171\tX=70298.20\ty=-33009.93 \nLabel=Strip\t172\tX=70653.36\ty=-32950.58 \nLabel=Strip\t173\tX=70309.49\ty=-32854.06 \nLabel=Strip\t174\tX=70664.63\ty=-32794.60 \nLabel=Strip\t175\tX=70320.73\ty=-32698.18 \nLabel=Strip\t176\tX=70675.85\ty=-32638.59 \nLabel=Strip\t177\tX=70331.92\ty=-32542.30 \nLabel=Strip\t178\tX=70687.02\ty=-32482.59 \nLabel=Strip\t179\tX=70343.06\ty=-32386.42 \nLabel=Strip\t180\tX=70698.13\ty=-32326.58 \nLabel=Strip\t181\tX=70354.14\ty=-32230.53 \nLabel=Strip\t182\tX=70709.20\ty=-32170.57 \nLabel=Strip\t183\tX=70365.17\ty=-32074.64 \nLabel=Strip\t184\tX=70720.20\ty=-32014.55 \nLabel=Strip\t185\tX=70376.14\ty=-31918.74 \nLabel=Strip\t186\tX=70731.16\ty=-31858.53 \nLabel=Strip\t187\tX=70387.06\ty=-31762.84 \nLabel=Strip\t188\tX=70742.06\ty=-31702.51 \nLabel=Strip\t189\tX=70397.93\ty=-31606.93 \nLabel=Strip\t190\tX=70752.90\ty=-31546.48 \nLabel=Strip\t191\tX=70408.74\ty=-31451.02 \nLabel=Strip\t192\tX=70763.70\ty=-31390.44 \nLabel=Strip\t193\tX=70419.50\ty=-31295.10 \nLabel=Strip\t194\tX=70774.44\ty=-31234.40 \nLabel=Strip\t195\tX=70430.21\ty=-31139.18 \nLabel=Strip\t196\tX=70785.12\ty=-31078.36 \nLabel=Strip\t197\tX=70440.87\ty=-30983.25 \nLabel=Strip\t198\tX=70795.76\ty=-30922.31 \nLabel=Strip\t199\tX=70451.47\ty=-30827.32 \nLabel=Strip\t200\tX=70806.34\ty=-30766.25 \nLabel=Strip\t201\tX=70462.01\ty=-30671.38 \nLabel=Strip\t202\tX=70816.86\ty=-30610.19 \nLabel=Strip\t203\tX=70472.51\ty=-30515.44 \nLabel=Strip\t204\tX=70827.34\ty=-30454.13 \nLabel=Strip\t205\tX=70482.95\ty=-30359.49 \nLabel=Strip\t206\tX=70837.76\ty=-30298.06 \nLabel=Strip\t207\tX=70493.33\ty=-30203.54 \nLabel=Strip\t208\tX=70848.12\ty=-30141.99 \nLabel=Strip\t209\tX=70503.67\ty=-30047.59 \nLabel=Strip\t210\tX=70858.44\ty=-29985.91 \nLabel=Strip\t211\tX=70513.95\ty=-29891.63 \nLabel=Strip\t212\tX=70868.69\ty=-29829.83 \nLabel=Strip\t213\tX=70524.18\ty=-29735.66 \nLabel=Strip\t214\tX=70878.90\ty=-29673.74 \nLabel=Strip\t215\tX=70534.35\ty=-29579.70 \nLabel=Strip\t216\tX=70889.05\ty=-29517.65 \nLabel=Strip\t217\tX=70544.47\ty=-29423.72 \nLabel=Strip\t218\tX=70899.15\ty=-29361.56 \nLabel=Strip\t219\tX=70554.53\ty=-29267.75 \nLabel=Strip\t220\tX=70909.20\ty=-29205.46 \nLabel=Strip\t221\tX=70564.55\ty=-29111.76 \nLabel=Strip\t222\tX=70919.19\ty=-29049.35 \nLabel=Strip\t223\tX=70574.51\ty=-28955.78 \nLabel=Strip\t224\tX=70929.13\ty=-28893.24 \nLabel=Strip\t225\tX=70584.41\ty=-28799.79 \nLabel=Strip\t226\tX=70939.01\ty=-28737.13 \nLabel=Strip\t227\tX=70594.27\ty=-28643.79 \nLabel=Strip\t228\tX=70948.84\ty=-28581.01 \nLabel=Strip\t229\tX=70604.07\ty=-28487.79 \nLabel=Strip\t230\tX=70958.62\ty=-28424.89 \nLabel=Strip\t231\tX=70613.81\ty=-28331.79 \nLabel=Strip\t232\tX=70968.34\ty=-28268.77 \nLabel=Strip\t233\tX=70623.50\ty=-28175.78 \nLabel=Strip\t234\tX=70978.01\ty=-28112.64 \nLabel=Strip\t235\tX=70633.14\ty=-28019.77 \nLabel=Strip\t236\tX=70987.63\ty=-27956.50 \nLabel=Strip\t237\tX=70642.73\ty=-27863.75 \nLabel=Strip\t238\tX=70997.19\ty=-27800.36 \nLabel=Strip\t239\tX=70652.26\ty=-27707.73 \nLabel=Strip\t240\tX=71006.70\ty=-27644.22 \nLabel=Strip\t241\tX=70661.74\ty=-27551.70 \nLabel=Strip\t242\tX=71016.16\ty=-27488.07 \nLabel=Strip\t243\tX=70671.16\ty=-27395.67 \nLabel=Strip\t244\tX=71025.56\ty=-27331.92 \nLabel=Strip\t245\tX=70680.53\ty=-27239.64 \nLabel=Strip\t246\tX=71034.91\ty=-27175.76 \nLabel=Strip\t247\tX=70689.85\ty=-27083.60 \nLabel=Strip\t248\tX=71044.21\ty=-27019.60 \nLabel=Strip\t249\tX=70699.12\ty=-26927.56 \nLabel=Strip\t250\tX=71053.45\ty=-26863.44 \nLabel=Strip\t251\tX=70708.33\ty=-26771.51 \nLabel=Strip\t252\tX=71062.64\ty=-26707.27 \nLabel=Strip\t253\tX=70717.49\ty=-26615.46 \nLabel=Strip\t254\tX=71071.78\ty=-26551.09 \nLabel=Strip\t255\tX=70726.59\ty=-26459.40 \nLabel=Strip\t256\tX=71080.86\ty=-26394.92 \nLabel=Strip\t257\tX=70735.64\ty=-26303.34 \nLabel=Strip\t258\tX=71089.89\ty=-26238.73 \nLabel=Strip\t259\tX=70744.64\ty=-26147.28 \nLabel=Strip\t260\tX=71098.86\ty=-26082.55 \nLabel=Strip\t261\tX=70753.58\ty=-25991.21 \nLabel=Strip\t262\tX=71107.79\ty=-25926.36 \nLabel=Strip\t263\tX=70762.47\ty=-25835.14 \nLabel=Strip\t264\tX=71116.65\ty=-25770.16 \nLabel=Strip\t265\tX=70771.31\ty=-25679.07 \nLabel=Strip\t266\tX=71125.47\ty=-25613.97 \nLabel=Strip\t267\tX=70780.09\ty=-25522.99 \nLabel=Strip\t268\tX=71134.23\ty=-25457.76 \nLabel=Strip\t269\tX=70788.82\ty=-25366.90 \nLabel=Strip\t270\tX=71142.94\ty=-25301.56 \nLabel=Strip\t271\tX=70797.50\ty=-25210.81 \nLabel=Strip\t272\tX=71151.59\ty=-25145.35 \nLabel=Strip\t273\tX=70806.12\ty=-25054.72 \nLabel=Strip\t274\tX=71160.19\ty=-24989.14 \nLabel=Strip\t275\tX=70814.69\ty=-24898.63 \nLabel=Strip\t276\tX=71168.74\ty=-24832.92 \nLabel=Strip\t277\tX=70823.21\ty=-24742.53 \nLabel=Strip\t278\tX=71177.23\ty=-24676.69 \nLabel=Strip\t279\tX=70831.68\ty=-24586.17 \nLabel=Strip\t280\tX=71185.67\ty=-24520.47 \nLabel=Strip\t281\tX=70840.08\ty=-24430.32 \nLabel=Strip\t282\tX=71194.06\ty=-24364.24 \nLabel=Strip\t283\tX=70848.43\ty=-24274.20 \nLabel=Strip\t284\tX=71202.39\ty=-24208.01 \nLabel=Strip\t285\tX=70856.73\ty=-24118.09 \nLabel=Strip\t286\tX=71210.67\ty=-24051.77 \nLabel=Strip\t287\tX=70864.98\ty=-23961.97 \nLabel=Strip\t288\tX=71218.89\ty=-23895.53 \nLabel=Strip\t289\tX=70873.18\ty=-23805.85 \nLabel=Strip\t290\tX=71227.07\ty=-23739.28 \nLabel=Strip\t291\tX=70881.32\ty=-23649.72 \nLabel=Strip\t292\tX=71235.18\ty=-23583.03 \nLabel=Strip\t293\tX=70889.41\ty=-23493.59 \nLabel=Strip\t294\tX=71243.25\ty=-23426.78 \nLabel=Strip\t295\tX=70897.44\ty=-23337.45 \nLabel=Strip\t296\tX=71251.26\ty=-23270.52 \nLabel=Strip\t297\tX=70905.42\ty=-23181.31 \nLabel=Strip\t298\tX=71259.22\ty=-23114.26 \nLabel=Strip\t299\tX=70913.35\ty=-23025.17 \nLabel=Strip\t300\tX=71267.12\ty=-22958.00 \nLabel=Strip\t301\tX=70921.22\ty=-22869.03 \nLabel=Strip\t302\tX=71274.97\ty=-22801.73 \nLabel=Strip\t303\tX=70929.04\ty=-22712.88 \nLabel=Strip\t304\tX=71282.77\ty=-22645.46 \nLabel=Strip\t305\tX=70936.81\ty=-22556.72 \nLabel=Strip\t306\tX=71290.51\ty=-22489.18 \nLabel=Strip\t307\tX=70944.52\ty=-22400.57 \nLabel=Strip\t308\tX=71298.20\ty=-22332.90 \nLabel=Strip\t309\tX=70952.18\ty=-22244.41 \nLabel=Strip\t310\tX=71305.84\ty=-22176.62 \nLabel=Strip\t311\tX=70959.79\ty=-22088.24 \nLabel=Strip\t312\tX=71313.42\ty=-22020.34 \nLabel=Strip\t313\tX=70967.34\ty=-21932.07 \nLabel=Strip\t314\tX=71320.95\ty=-21864.05 \nLabel=Strip\t315\tX=70974.84\ty=-21775.90 \nLabel=Strip\t316\tX=71328.43\ty=-21707.75 \nLabel=Strip\t317\tX=70982.28\ty=-21619.73 \nLabel=Strip\t318\tX=71335.85\ty=-21551.46 \nLabel=Strip\t319\tX=70989.68\ty=-21463.55 \nLabel=Strip\t320\tX=71343.22\ty=-21395.15 \nLabel=Strip\t321\tX=70997.01\ty=-21307.37 \nLabel=Strip\t322\tX=71350.53\ty=-21238.85 \nLabel=Strip\t323\tX=71004.30\ty=-21151.18 \nLabel=Strip\t324\tX=71357.79\ty=-21082.54 \nLabel=Strip\t325\tX=71011.53\ty=-20994.99 \nLabel=Strip\t326\tX=71365.00\ty=-20926.23 \nLabel=Strip\t327\tX=71018.71\ty=-20838.80 \nLabel=Strip\t
